vi "Write Resample Vector Table to BRAM from Host.vi"(7 "Resample Table":refnum<k21>="Resample Vector Table", 8 "Write?":bool, 10 "Data":T1 {"x[n].ResampleInfo"."Lambda" format="%.18g"; "x[n-1].ResampleInfo"."Lambda" format="%.18g"}, 11 "Address":u16) -> ()   [LabVIEW 2011]
uses:
  <vilib>/rvi/DataTransferAndStorage/Container/Common/niFpgaContainerExecOnDevCompGetState.vi
  <vilib>/rvi/Memory/Memory_Emulation/niFpgaMemoryEmulationValidateCache.vi
  <vilib>/rvi/DataTransferAndStorage/Container/Common/niFpgaContainerGetUniqueNameForEmu.vi
  <vilib>/rvi/Memory/Memory_Emulation/nirvimemoryEmulationManagerCache_InsertValue.vi
  <vilib>/Utility/error.llb/Clear Errors.vi
  <vilib>/rvi/Memory/Memory_Emulation/nirvimemoryEmulationManagerCache_GetValue.vi
  <vilib>/rvi/Memory/Memory_Emulation/nirvimemoryEmulationManagerCache_SetValue.vi
  <vilib>/rvi/FXPMathLib/basic elements/FxpDiscreteDelay/XNode/nifxpmath_DiscreteDelay.xnode
  <vilib>/rvi/DataTransferAndStorage/Container/XNode/niFpgaContainer.xnode
  <vilib>/rvi/Memory/Memory_Emulation/niFpgaMemoryEmulationRefIn.vi
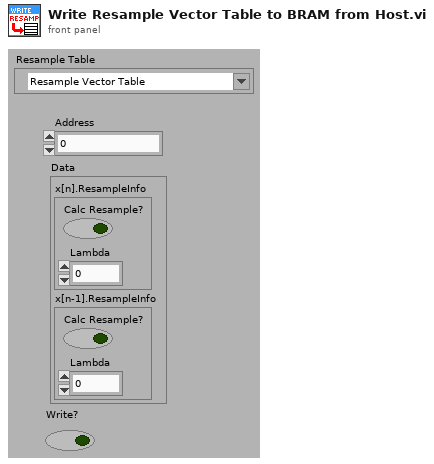
[diagram p1: front panel]
types:
  T1 = cluster{"x[n].ResampleInfo":cluster{"Calc Resample?":bool, "Lambda":fxp<+/-,18,1>}, "x[n-1].ResampleInfo":cluster{"Calc Resample?":bool, "Lambda":fxp<+/-,18,1>}}
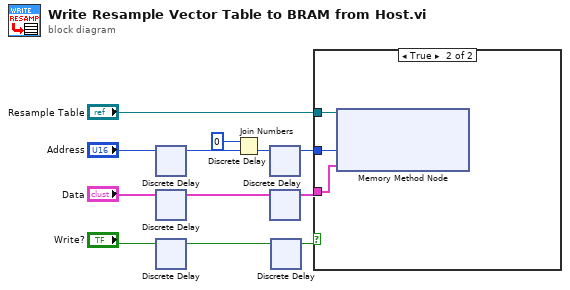
[diagram p0: block diagram]
diagram:
  n1 = xnode "Discrete Delay"("D"="Address") -> ("Q"=w6:u16)
  n2 = xnode "Discrete Delay"("D"="Data") -> ("Q"=w5:T1)
  n3 = xnode "Discrete Delay"("D"="Write?") -> ("Q"=w4:bool)
  n4 = Join Numbers(hi=u16 0, lo=w6) -> ((hi.lo)=w8:u32)
  n5 = xnode "Discrete Delay"("D"=w8) -> ("Q"=w3:u32)
  n6 = xnode "Discrete Delay"("D"=w5) -> ("Q"=w2:T1)
  n7 = xnode "Discrete Delay"("D"=w4) -> ("Q"=w1:bool)
  n8 = case shown="True" w1 {
    tunnel: "Resample Table" -> [_ w15]
    tunnel: w3 -> [_ w14]
    tunnel: w2 -> [_ w13]
    frame False {
    }
    frame True {
      n9 = xnode ("Memory Method Node")("Address"=w14, "Data"=w13, "Memory In"=w15) -> ()  [unwired: 1 out]
    }
  }
